vi "set_dc_voltage.vi"(8 "error in (no error)":errorcluster, 10 "motech_set_value":T4, 11 "UI in":T1) -> (0 "error out":errorcluster, 3 "UI out 2":T1)   [LabVIEW 2017]
uses:
  motech_power_supply/types/motech_set_value_cluster.ctl
  motech_power_supply/types/channels_enum.ctl
  ui.ctl
  classes/dc_power_supply/DC_power_supply.lvclass
  classes/report/Report.lvclass
  ui_buttons.ctl
  types/boc_type.ctl
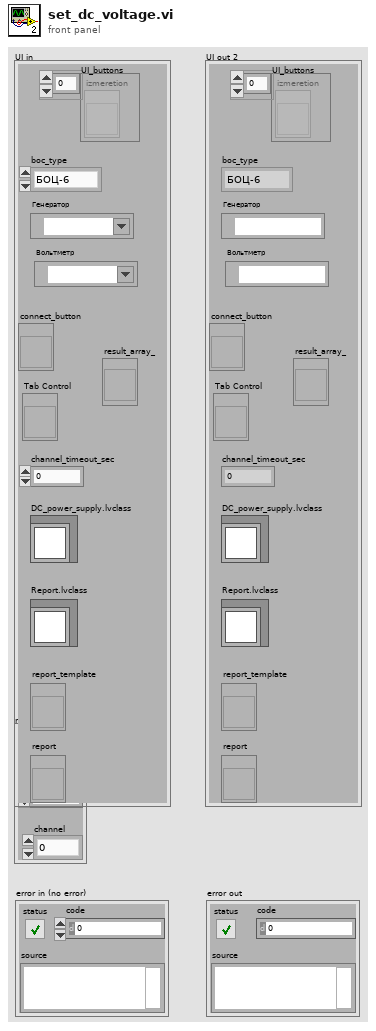
[diagram p1: front panel]
types:
  T1 = typedef "ui.ctl" = cluster{"UI_buttons":T2, "Tab Control":refnum<vi>, "connect_button":refnum<vi>, "generator":refnum<visa-resource-name>, "voltmetr":refnum<visa-resource-name>, "channel_timeout_sec":dbl, "boc_type":T3, "result_array_":refnum<vi>, "DC_power_supply.lvclass":refnum<class "DC_power_supply.lvclass">, "Report.lvclass":refnum<class "Report.lvclass">, "report_template":refnum<vi>, "report":refnum<vi>}
  T2 = typedef "ui_buttons.ctl" = refnum<vi>[]
  T3 = typedef "boc_type.ctl" = enum16{"БОЦ-6", "БОЦ-12"}
  T4 = typedef "motech_set_value_cluster.ctl" = cluster{"voltage":dbl, "current":dbl, "channel":T5}
  T5 = typedef "channels_enum.ctl" = enum16{"0", "1", "2"}
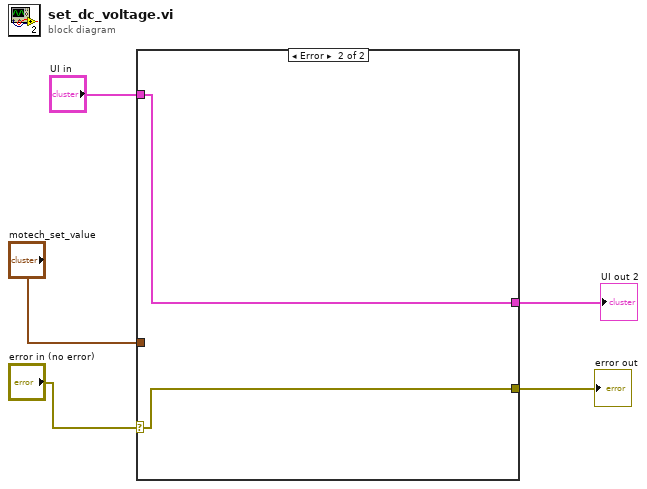
[diagram p0: block diagram]
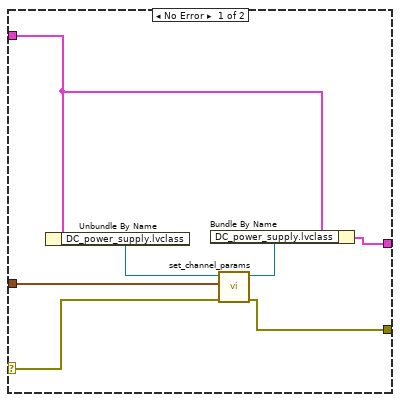
[diagram p2: hidden frame]
diagram:
  n1 = case shown="Error" "error in (no error)" {
    selector: "error in (no error)" -> [w6 w13]
    tunnel: "motech_set_value" -> [w12 _]
    tunnel: [w11 w13] -> w4
    tunnel: "UI in" -> [w10 w14]
    tunnel: [w9 w14] -> w2
    frame No Error {
      n2 = Unbundle By Name(w10) -> ("DC_power_supply.lvclass"=w7:refnum<class "DC_power_supply.lvclass">)
      n3 = call-dynamic "set_channel_params.vi"("error in (no error)"=w6, "motech_set_value"=w12, "DC_power_supply in"=w7) -> ("error out"=w11:errorcluster, "DC_power_supply out"=w8:refnum<class "DC_power_supply.lvclass">)  [unwired: 7 in]
      n4 = Bundle By Name(cluster=w10, "DC_power_supply.lvclass"=w8) -> (w9:T1)
    }
    frame Error {
    }
  }
  "error out" <- w4
  "UI out 2" <- w2
